vi "Main_Old.vi"() -> ()   [LabVIEW 2023]
uses:
  System states.ctl
  System variables.ctl
  <vilib>/Utility/file.llb/Read Delimited Spreadsheet (string).vi
  <vilib>/Utility/file.llb/Write Delimited Spreadsheet (string).vi
  Numato/Numato.lvlib
  DO_Reley/DO_Relay.lvlib
panel:
  in  "Tab Control":T1(tab)
  in  "Login":bool
  in  "Lozinka":string
  in  "Dostupne varijante":string(combo)
  in  "Select Variant":bool=TRUE
  in  "Izabrana varijanta":string
  in  "Cassete numbers":map{string, i32}(c390)
  out "Variants->FileNames":map{string, string}(c390)
  in  "Serial number":string
  in  "Report Erase":bool
  in  "START":bool
  in  "Status":bool[](array[boolean])
  in  "Stop":bool
  out "Monitor":string
  # "Rezultat brisanja programa :"
  # "Serisjki broj za brisanje :"
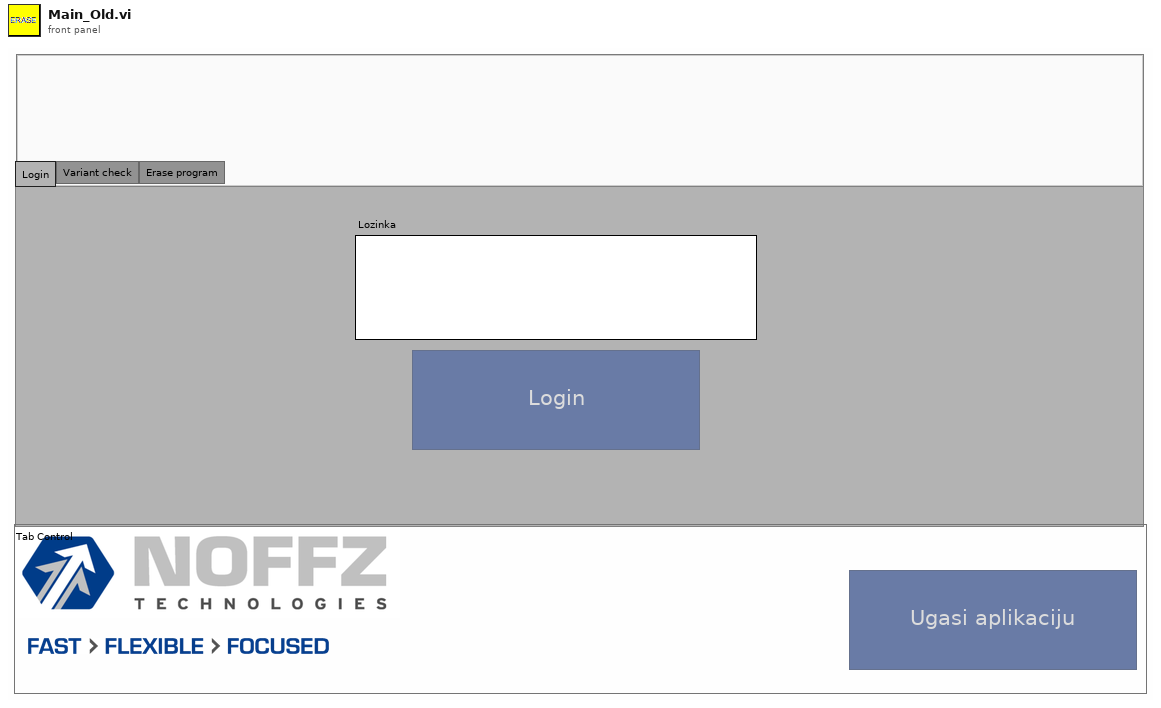
[diagram p1: front panel]
types:
  T1 = enum32{"Login", "Variant check", "Erase program"}
  T2 = typedef "System variables.ctl" = cluster{"Relay 1":refnum<visa-resource-name>, "Relay 2":refnum<visa-resource-name>, "Releji":cluster{"Vdd":i32, "GND":i32, "PGD":i32, "PGC":i32, "Reset":i32, "Reference":refnum<visa-resource-name>}, "DUT1":bool, "Family name":string, "DUT 2":bool, "DUT test?":bool, "DI0-7":i32, "DI8-15":i32, "DO0-8":i32, "References":cluster{"Relays":bool, "DIO":bool}}
  T3 = typedef "System states.ctl" = enum16{"Login", "Check Variant", "Dispaly variants", "Correct Variant", "Incorrect variant", "Initialize", "Check present boards", "Idle", "Connect relays", "Erasing", "Disconnect relays", "Erase Finished", "Deinitialize", "Erase report", "Set variables"}
  T4 = cluster{"Vdd":i32, "GND":i32, "PGD":i32, "PGC":i32, "Reset":i32, "Reference":refnum<visa-resource-name>}
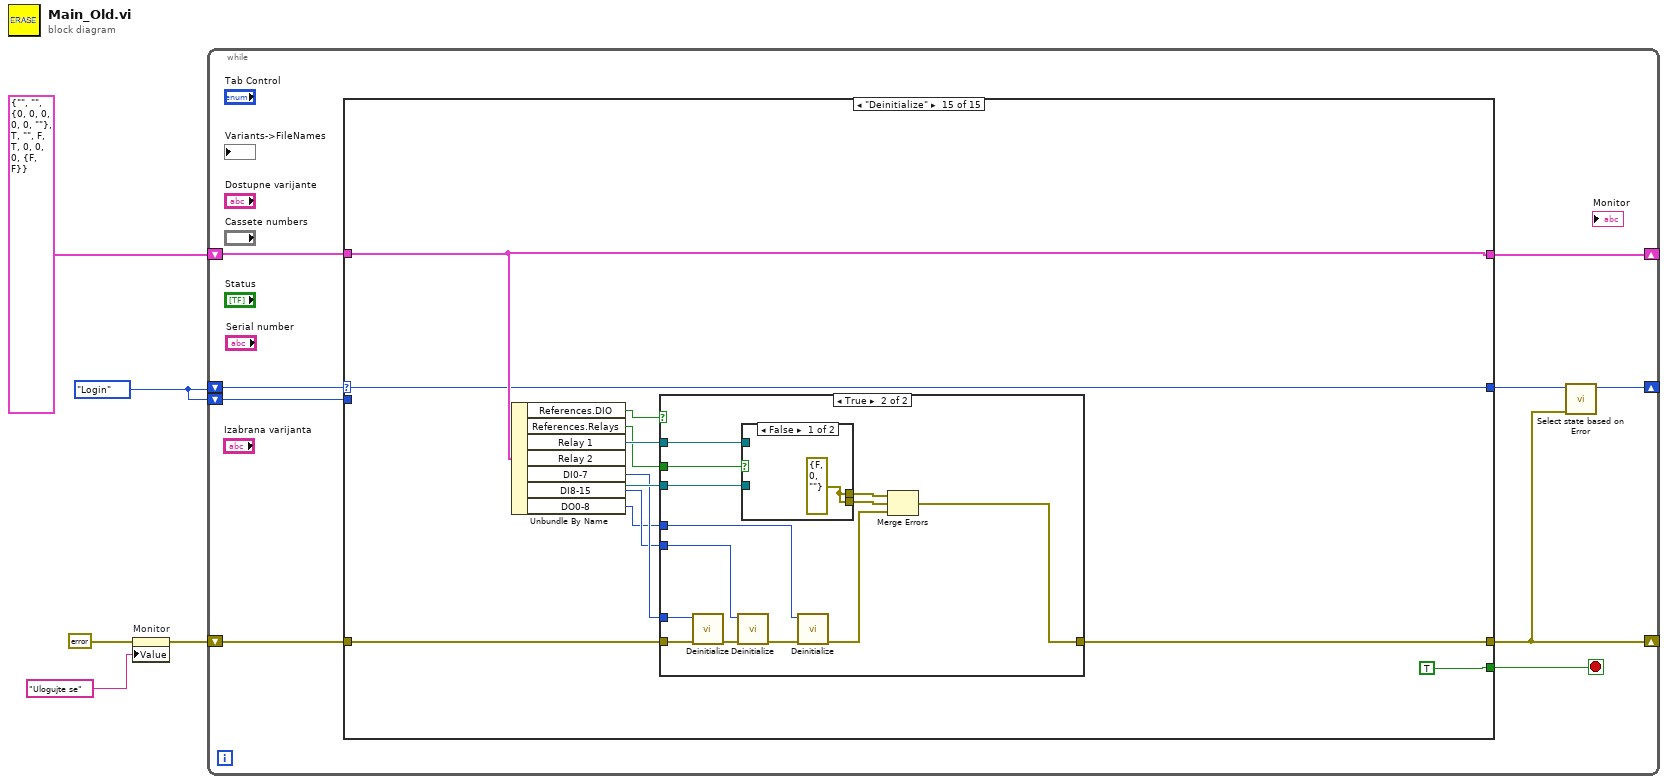
[diagram p0: block diagram]
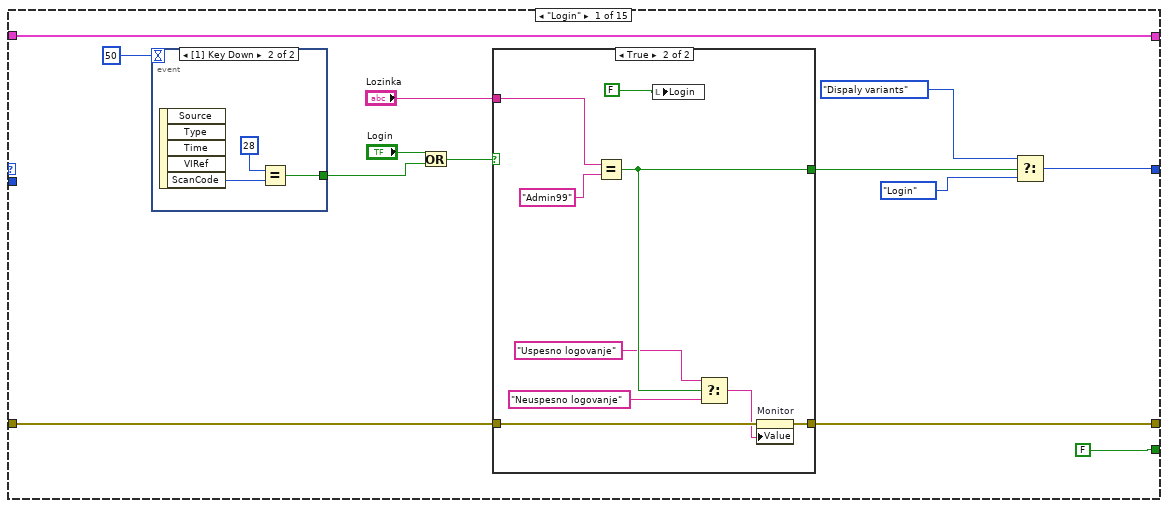
[diagram p2: hidden frame]
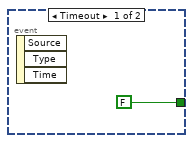
[diagram p3: hidden frame]
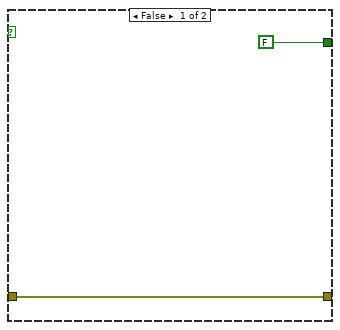
[diagram p4: hidden frame]
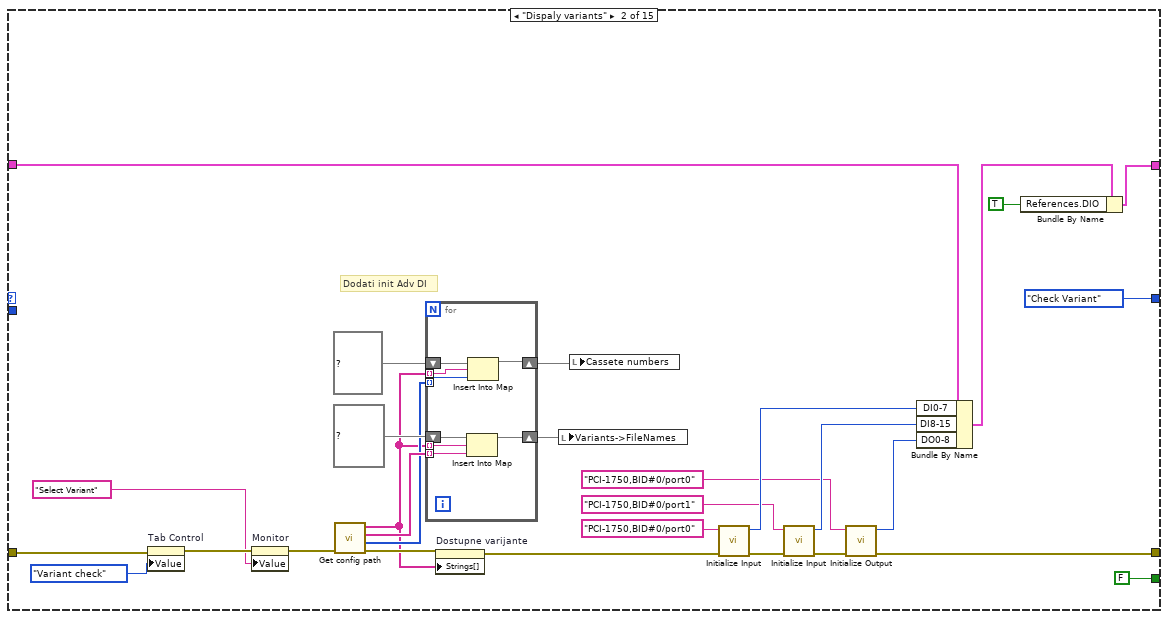
[diagram p5: hidden frame]
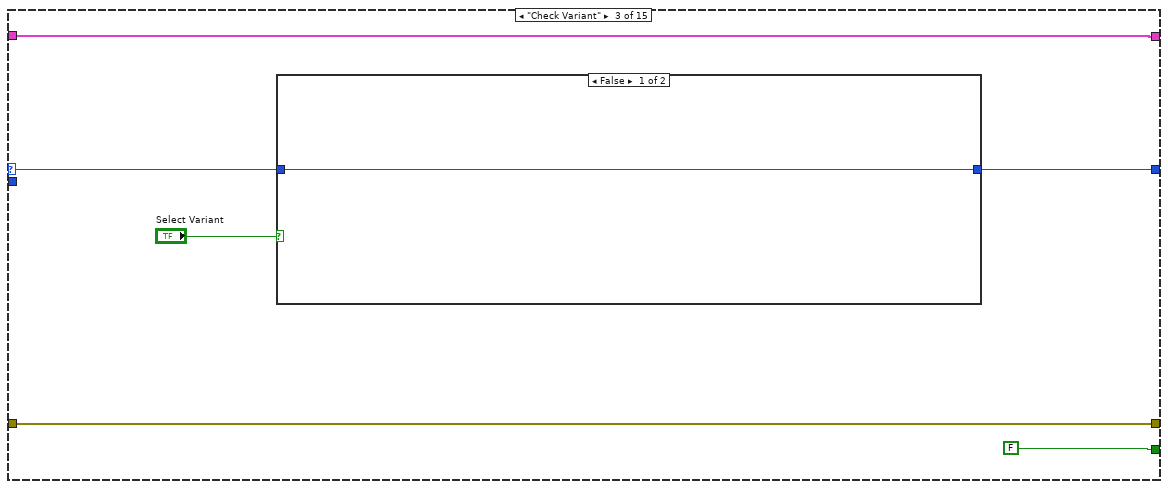
[diagram p6: hidden frame]
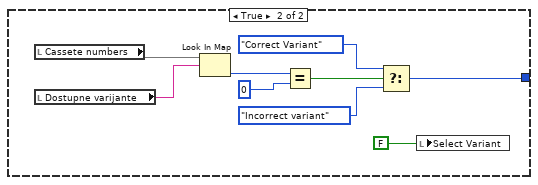
[diagram p7: hidden frame]
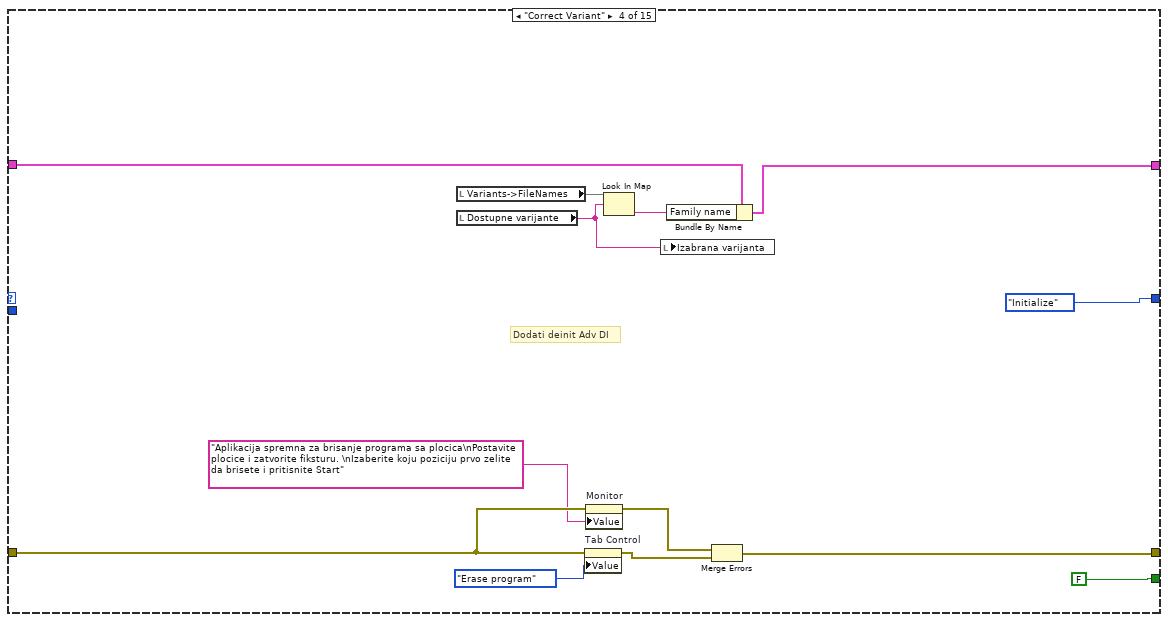
[diagram p8: hidden frame]
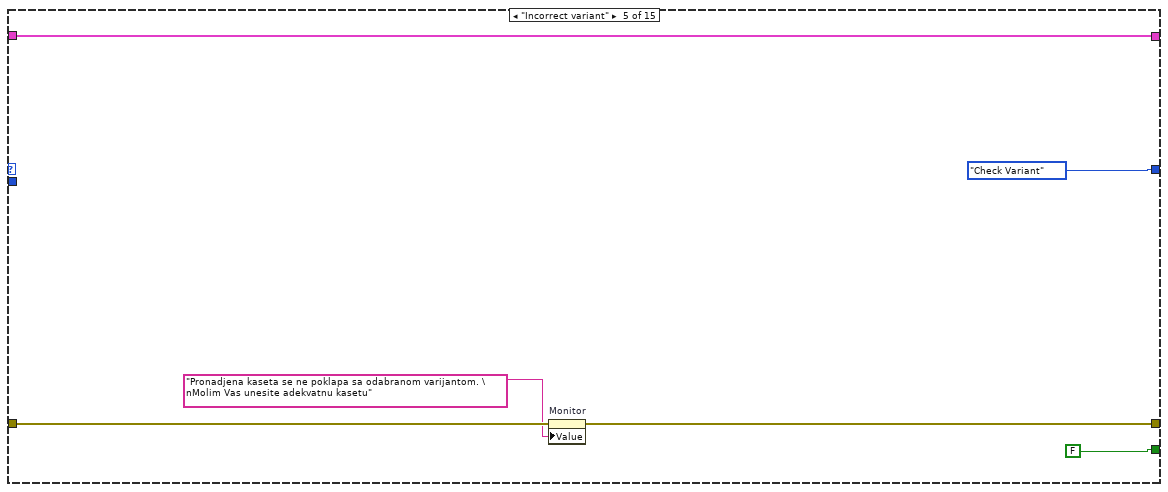
[diagram p9: hidden frame]
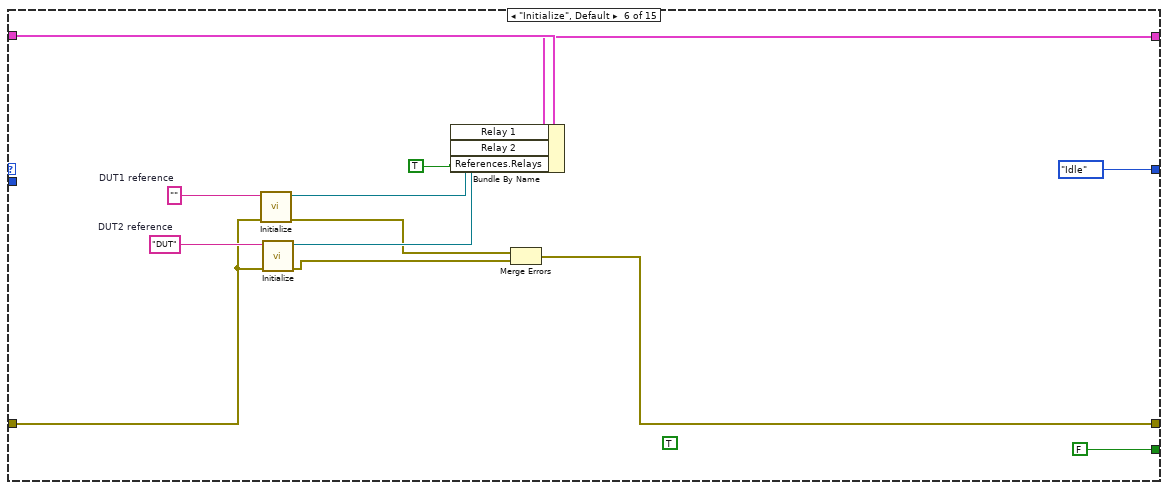
[diagram p10: hidden frame]
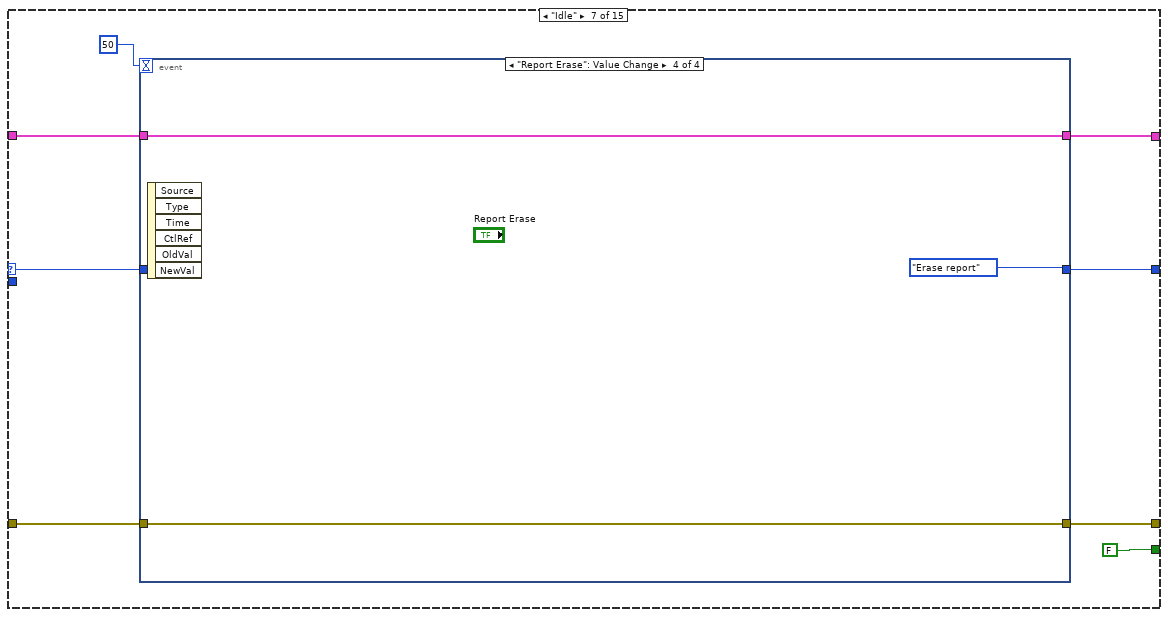
[diagram p11: hidden frame]
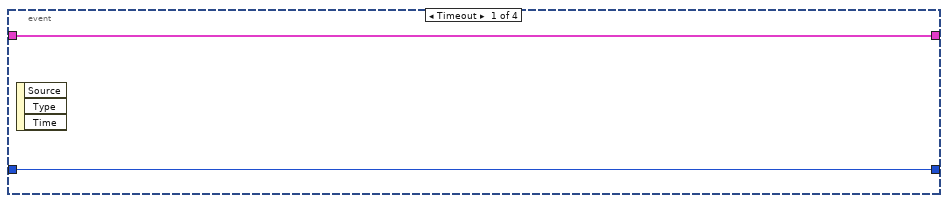
[diagram p12: hidden frame]
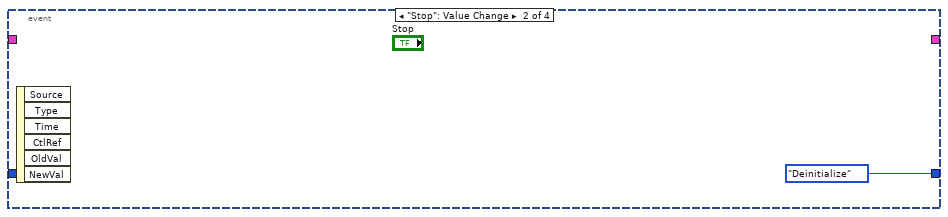
[diagram p13: hidden frame]
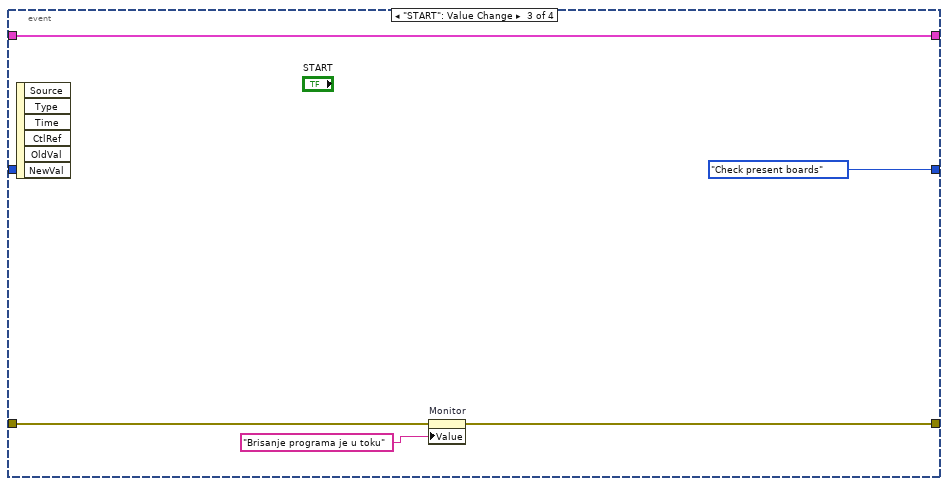
[diagram p14: hidden frame]
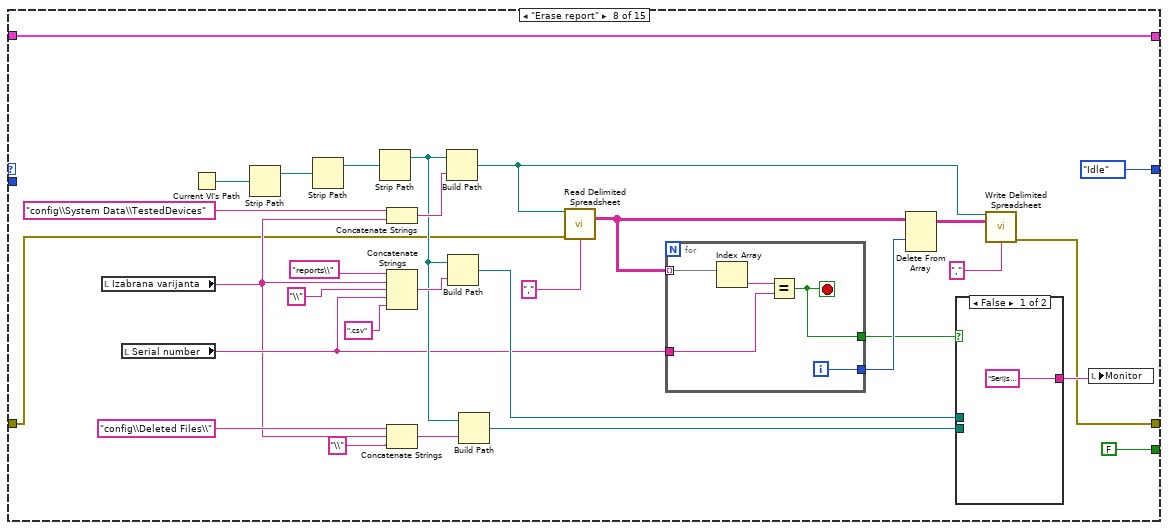
[diagram p15: hidden frame]
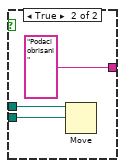
[diagram p16: hidden frame]
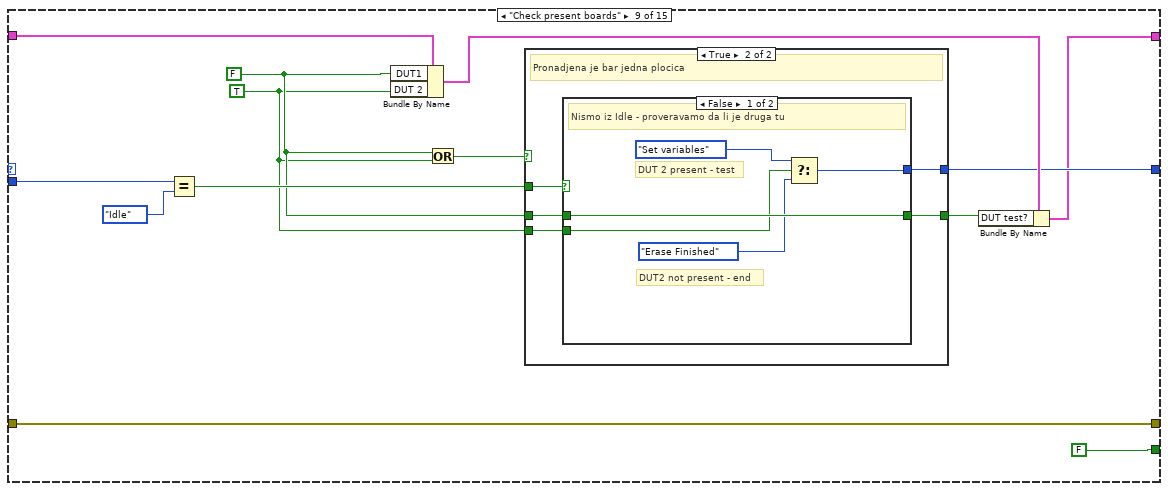
[diagram p17: hidden frame]
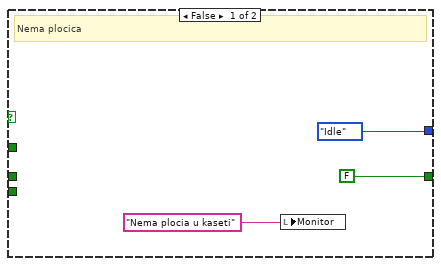
[diagram p18: hidden frame]
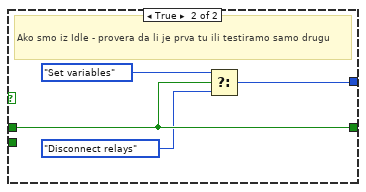
[diagram p19: hidden frame]
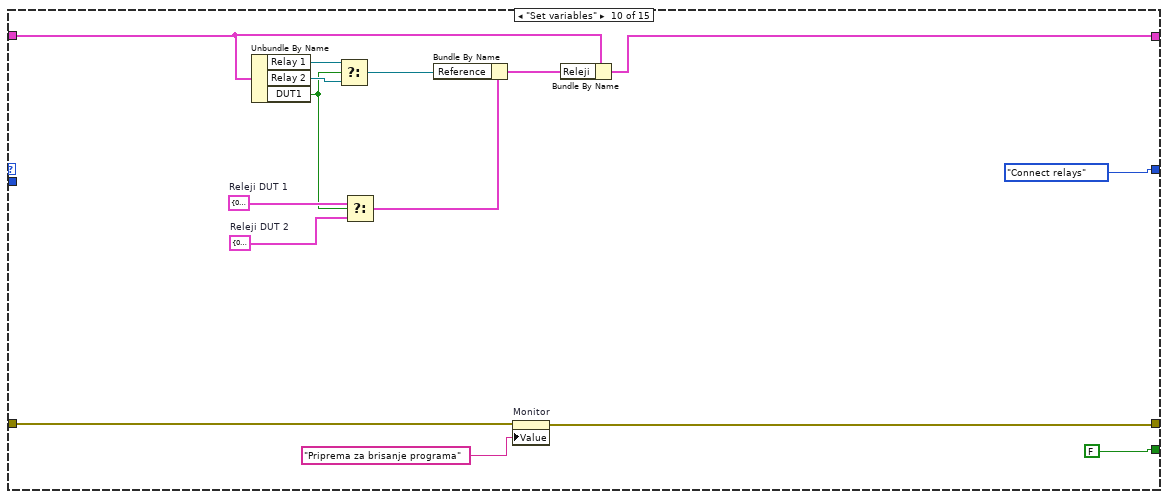
[diagram p20: hidden frame]
diagram:
  w1 = System_states."Login"
  n1 = property on="Monitor" class="Str"(error in=errorcluster {"status"=FALSE, "code"=0, "source"=""} ("error in (no error)"), "Value"="Ulogujte se" ("Monitor")) -> (error out=w3:errorcluster)  [unwired: 1 in, 1 out]
  n2 = while {
    shift-right: [w9] -> _
    shift-left: T2 {"Relay 1"="", "Relay 2"="", "Releji"={"Vdd"=0, "GND"=0, "PGD"=0, "PGC"=0, "Reset"=0, "Reference"=""}, "DUT1"=TRUE, "Family name"="", "DUT 2"=FALSE, "DUT test?"=TRUE, "DI0-7"=0, "DI8-15"=0, "DO0-8"=0, "References"={"Relays"=FALSE, "DIO"=FALSE}} -> [w13]
    shift-right: [w10] -> _
    shift-left: w3 -> [w14]
    shift-right: [w11] -> _
    shift-left: w1 -> [w7]
    shift-left: w1 -> [w6]
    stop <- w8 stop-if-true
    n3 = case shown="\"Deinitialize\"" w7 {
      selector: w7 -> [_ _ w84 _ _ _ w131 _ _ _ _ _ _ _ w278]
      tunnel: w14 -> [w21 w70 w82 w101 w114 w125 w129 w151 w195 w219 w235 w249 w262 w268 w276]
      tunnel: w13 -> [w15 w54 w80 w103 w111 w124 w134 w147 w198 w226 w234 w244 w259 w269 w280]
      tunnel: [w15 w44 w80 w102 w111 w123 w133 w147 w187 w230 w234 w244 w259 w269 w280] -> w9
      tunnel: [w20 w51 w82 w100 w113 w116 w128 w150 w195 w218 w236 w247 w261 w267 w275] -> w10
      tunnel: [w25 System_states."Check Variant" w83 System_states."Initialize" System_states."Check Variant" System_states."Idle" w132 System_states."Idle" w196 System_states."Connect relays" System_states."Erasing" System_states."Disconnect relays" w255 System_states."Idle" w278] -> w12
      tunnel: [FALSE ("Boolean") FALSE ("Boolean") FALSE ("Boolean") FALSE ("Boolean") FALSE ("Boolean") FALSE ("Boolean") FALSE ("Boolean") FALSE ("Boolean") FALSE ("Boolean") FALSE ("Boolean") FALSE ("Boolean") FALSE ("Boolean") FALSE ("Boolean") FALSE ("Boolean") TRUE ("Boolean")] -> w8
      tunnel: w6 -> [_ _ _ _ _ _ _ _ w193 _ _ _ _ _ _]
      frame "Login" {
        n4 = event shown="[1] Key Down" {
          selector: _ -> [_ _]
          dyn-events: _ -> [_ _]
          timeout: 50 -> [_ _]
          tunnel: [FALSE w29] -> w18
          event Timeout {
            n5 = event-data() -> ()  [unwired: 1 in, 3 out]
          }
          event Key Down {
            n6 = event-data() -> ("ScanCode"=w31:i16)  [unwired: 1 in, 4 out]
            n7 = Equal?(x=i16 28, y=w31) -> (x = y?=w29:bool)
          }
        }
        n8 = Or(x="Login", y=w18) -> (x .or. y?=w17:bool)
        n9 = case shown="True" w17 {
          tunnel: "Lozinka" -> [_ w42]
          tunnel: [FALSE w37] -> w22
          tunnel: w21 -> [w32 w39]
          tunnel: [w32 w38] -> w20
          frame False {
          }
          frame True {
            n10 = Equal?(x=w42, y="Admin99") -> (x = y?=w37:bool)
            n11 = local write "Login"(FALSE ("Login")) -> ()
            n12 = Select(t="Uspesno logovanje" ("y"), s=w37, f="Neuspesno logovanje" ("y")) -> (s? t:f=w34:string)
            n13 = property on="Monitor" class="Str"(error in=w39, "Value"=w34) -> (error out=w38:errorcluster)  [unwired: 1 in, 1 out]
          }
        }
        n14 = Select(t=System_states."Dispaly variants", s=w22, f=System_states."Login") -> (s? t:f=w25:T3)
      }
      frame "Dispaly variants" {
        # "Dodati init Adv DI"
        n15 = property on="Tab Control" class="TabCtl (strict)"(error in=w70, "Value"=T1."Variant check" ("Tab Control")) -> (error out=w68:errorcluster)  [unwired: 1 in, 1 out]
        n16 = property on="Monitor" class="Str"(error in=w68, "Value"="Select Variant" ("Monitor")) -> (error out=w66:errorcluster)  [unwired: 1 in, 1 out]
        n17 = call "Get config path.vi"("error in"=w66) -> ("error out"=w65:errorcluster, "Cassette codes"=w58:i32[], "Family names"=w64:string[], "Variants"=w57:string[])  [unwired: 7 in]
        n18 = for {
          tunnel: w57 -> [w77] mode=indexing
          tunnel: w64 -> [w76] mode=indexing
          shift-right: [w78] -> w61
          shift-left: map{string, string} {} ("Variants->FileNames") -> [w79]
          shift-right: [w74] -> w59
          shift-left: map{string, i32} {} ("map") -> [w75]
          tunnel: w57 -> [w73] mode=indexing
          tunnel: w58 -> [w72] mode=indexing
          n19 = Insert Into Map(map in=w79, key=w77, value=w76) -> (map out=w78:map{string, string})  [unwired: 2 out]
          n20 = Insert Into Map(map in=w75, key=w73, value=w72) -> (map out=w74:map{string, i32})  [unwired: 2 out]
        }
        n21 = property on="Dostupne varijante" class="CmbBox"(error in=w65, "Strings[]"=w57) -> (error out=w56:errorcluster)  [unwired: 1 in, 1 out]
        n22 = local write "Variants->FileNames"(w61) -> ()
        n23 = local write "Cassete numbers"(w59) -> ()
        n24 = call "Initialize Input.vi"("error in"=w56, "Physical channels in"="PCI-1750,BID#0/port0") -> ("error out"=w53:errorcluster, "task out"=w50:i32)  [unwired: 8 in]
        n25 = call "Initialize Input.vi"("error in"=w53, "Physical channels in"="PCI-1750,BID#0/port1") -> ("error out"=w52:errorcluster, "task out"=w49:i32)  [unwired: 8 in]
        n26 = call "Initialize Output.vi"("error in"=w52, "Physical channels in"="PCI-1750,BID#0/port0") -> ("error out"=w51:errorcluster, "task out"=w48:i32)  [unwired: 8 in]
        n27 = Bundle By Name(cluster=w54, "DI0-7"=w50, "DI8-15"=w49, "DO0-8"=w48) -> (w45:T2)
        n28 = Bundle By Name(cluster=w45, "References.DIO"=TRUE) -> (w44:T2)
      }
      frame "Check Variant" {
        n29 = case shown="False" "Select Variant" {
          tunnel: w84 -> [w86 _]
          tunnel: [w86 w93] -> w83
          frame False {
          }
          frame True {
            n30 = local read "Cassete numbers"() -> (w92:map{string, i32})
            n31 = local read "Dostupne varijante"() -> (w94:string)
            n32 = Look In Map(map=w92, key=w94) -> (value=w91:i32)  [unwired: 1 in, 1 out]
            n33 = Equal?(x=w91, y=0) -> (x = y?=w89:bool)
            n34 = Select(t=System_states."Correct Variant", s=w89, f=System_states."Incorrect variant") -> (s? t:f=w93:T3)
            n35 = local write "Select Variant"(FALSE ("Select Variant")) -> ()
          }
        }
      }
      frame "Correct Variant" {
        # "Dodati deinit Adv DI"
        n36 = local read "Variants->FileNames"() -> (w105:map{string, string})
        n37 = local read "Dostupne varijante"() -> (w96:string)
        n38 = property on="Tab Control" class="TabCtl (strict)"(error in=w101, "Value"=T1."Erase program" ("Tab Control")) -> (error out=w106:errorcluster)  [unwired: 1 in, 1 out]
        n39 = property on="Monitor" class="Str"(error in=w101, "Value"="Aplikacija spremna za brisanje programa sa plocica\nPostavite plocice i zatvorite fiksturu. \nIzaberite koju poziciju prvo zelite da brisete i pritisnite Start" ("Monitor")) -> (error out=w107:errorcluster)  [unwired: 1 in, 1 out]
        n40 = Look In Map(map=w105, key=w96) -> (value=w104:string)  [unwired: 1 in, 1 out]
        n41 = local write "Izabrana varijanta"(w96) -> ()
        n42 = Bundle By Name(cluster=w103, "Family name"=w104) -> (w102:T2)
        n43 = Merge Errors(w107, w106) -> (w100:errorcluster)
      }
      frame "Incorrect variant" {
        n44 = property on="Monitor" class="Str"(error in=w114, "Value"="Pronadjena kaseta se ne poklapa sa odabranom varijantom. \nMolim Vas unesite adekvatnu kasetu" ("Monitor")) -> (error out=w113:errorcluster)  [unwired: 1 in, 1 out]
      }
      frame "Initialize", Default {
        (unwired) TRUE ("DUT 1")
        w126 = ""  # DUT1 reference
        w127 = "DUT"  # DUT2 reference
        n45 = call "Initialize.vi"("error in (no error)"=w125, "Resource"=w126) -> ("error out"=w120:errorcluster, "VISA resource name out"=w122:refnum<visa-resource-name>)  [unwired: 8 in]
        n46 = call "Initialize.vi"("error in (no error)"=w125, "Resource"=w127) -> ("error out"=w119:errorcluster, "VISA resource name out"=w121:refnum<visa-resource-name>)  [unwired: 8 in]
        n47 = Bundle By Name(cluster=w124, "Relay 1"=w122, "Relay 2"=w121, "References.Relays"=TRUE) -> (w123:T2)
        n48 = Merge Errors(w120, w119) -> (w116:errorcluster)
      }
      frame "Idle" {
        n49 = event shown="[3] \"Report Erase\": Value Change" {
          selector: _ -> [_ _ _ _]
          dyn-events: _ -> [_ _ _ _]
          timeout: 50 -> [_ _ _ _]
          tunnel: w134 -> [w137 _ w142 w144]
          tunnel: [w137 _ w142 w144] -> w133
          tunnel: [w136 System_states."Deinitialize" System_states."Check present boards" System_states."Erase report"] -> w132
          tunnel: w131 -> [w136 _ _ _]
          tunnel: w129 -> [_ _ w141 w145]
          tunnel: [_ _ w140 w145] -> w128
          event Timeout {
            n50 = event-data() -> ()  [unwired: 1 in, 3 out]
          }
          event "Stop": Value Change {
            n51 = event-data() -> ()  [unwired: 1 in, 6 out]
          }
          event "START": Value Change {
            n52 = event-data() -> ()  [unwired: 1 in, 6 out]
            n53 = property on="Monitor" class="Str"(error in=w141, "Value"="Brisanje programa je u toku" ("Monitor")) -> (error out=w140:errorcluster)  [unwired: 1 in, 1 out]
          }
          event "Report Erase": Value Change {
            n54 = event-data() -> ()  [unwired: 1 in, 6 out]
          }
        }
      }
      frame "Erase report" {
        n55 = local read "Izabrana varijanta"() -> (w156:string)
        n56 = local read "Serial number"() -> (w158:string)
        n57 = Current VI's Path() -> (path=w174:path)
        n58 = Strip Path(path=w174) -> (stripped path=w175:path)  [unwired: 1 out]
        n59 = Strip Path(path=w175) -> (stripped path=w176:path)  [unwired: 1 out]
        n60 = Strip Path(path=w176) -> (stripped path=w163:path)  [unwired: 1 out]
        n61 = Concatenate Strings("config\\System Data\\TestedDevices", w156) -> (w172:string)
        n62 = Concatenate Strings("reports\\", w156, "\\" ("string"), w158, ".csv" ("string")) -> (w165:string)
        n63 = Concatenate Strings("config\\Deleted Files\\", w156, "\\" ("string")) -> (w161:string)
        n64 = Build Path(base path=w163, name or relative path=w172) -> (appended path=w167:path)
        n65 = Build Path(base path=w163, name or relative path=w165) -> (appended path=w164:path)
        n66 = Build Path(base path=w163, name or relative path=w161) -> (appended path=w154:path)
        n67 = call-poly <vilib>:"Read Delimited Spreadsheet.vi"("file path (dialog if empty)"=w167, "error in (no error)"=w151, "delimiter (\\t)"="," ("delimiter (\\t)")) -> ("all rows"=w170:string[][])  [unwired: 7 in, 5 out]
        n68 = for {
          tunnel: w170 -> [w185] mode=indexing
          tunnel: w158 -> [w183]
          tunnel: [w182] -> w169
          tunnel: [w181] -> w153
          i -> [w182]
          stop <- w181 stop-if-true
          n69 = Index Array(array=w185) -> (element=w184:string)  [unwired: 1 in]
          n70 = Equal?(x=w184, y=w183) -> (x = y?=w181:bool)
        }
        n71 = Delete From Array(array=w170, index (row)=w169) -> (array with subset deleted=w168:string[][])  [unwired: 2 in, 1 out]
        n72 = case shown="False" w153 {
          tunnel: w164 -> [_ w180]
          tunnel: w154 -> [_ w179]
          tunnel: ["Serijski broj nije pronajden u brojacu testiranja" ("Monitor") "Podaci obrisani" ("Monitor")] -> w152
          frame False {
          }
          frame True {
            n73 = Move(source path=w180, 10:w179) -> ()  [unwired: 3 in, 3 out]
          }
        }
        n74 = call-poly <vilib>:"Write Delimited Spreadsheet.vi"("file path (dialog if empty)"=w167, "2D data"=w168, "delimiter (\\t)"="," ("delimiter (\\t)")) -> ("error out"=w150:errorcluster)  [unwired: 11 in, 1 out]
        n75 = local write "Monitor"(w152) -> ()
      }
      frame "Check present boards" {
        w189 = FALSE ("DUT1")
        w188 = TRUE
        n76 = Equal?(x=w193, y=System_states."Idle") -> (x = y?=w191:bool)
        n77 = Bundle By Name(cluster=w198, "DUT1"=w189, "DUT 2"=w188) -> (w197:T2)
        n78 = Or(x=w189, y=w188) -> (x .or. y?=w190:bool)
        n79 = case shown="True" w190 {
          tunnel: [System_states."Idle" ("f") w206] -> w196
          tunnel: w191 -> [_ w205]
          tunnel: w189 -> [_ w204]
          tunnel: w188 -> [_ w203]
          tunnel: [FALSE ("DUT1") w202] -> w186
          frame False {
            # "Nema plocica"
            n80 = local write "Monitor"("Nema plocia u kaseti" ("Monitor")) -> ()
          }
          frame True {
            # "Pronadjena je bar jedna plocica"
            n81 = case shown="False" w205 {
              tunnel: [w208 w214] -> w206
              tunnel: w204 -> [w211 w215]
              tunnel: w203 -> [w210 _]
              tunnel: [w211 w215] -> w202
              frame False {
                # "DUT2 not present - end"
                # "DUT 2 present - test"
                # "Nismo iz Idle - proveravamo da li je druga tu"
                n82 = Select(t=System_states."Set variables", s=w210, f=System_states."Erase Finished") -> (s? t:f=w208:T3)
              }
              frame True {
                # "Ako smo iz Idle - provera da li je prva tu ili testiramo samo drugu"
                n83 = Select(t=System_states."Set variables" ("f"), s=w215, f=System_states."Disconnect relays") -> (s? t:f=w214:T3)
              }
            }
          }
        }
        n84 = Bundle By Name(cluster=w197, "DUT test?"=w186) -> (w187:T2)
      }
      frame "Set variables" {
        w228 = T4 {"Vdd"=0, "GND"=0, "PGD"=0, "PGC"=0, "Reset"=0, "Reference"=""}  # Releji DUT 2
        w229 = T4 {"Vdd"=0, "GND"=0, "PGD"=0, "PGC"=0, "Reset"=0, "Reference"=""}  # Releji DUT 1
        n85 = Unbundle By Name(w226) -> ("Relay 1"=w225:refnum<visa-resource-name>, "Relay 2"=w224:refnum<visa-resource-name>, "DUT1"=w220:bool)
        n86 = Select(t=w225, s=w220, f=w224) -> (s? t:f=w223:refnum<visa-resource-name>)
        n87 = Select(t=w229, s=w220, f=w228) -> (s? t:f=w227:T4)
        n88 = Bundle By Name(cluster=w227, "Reference"=w223) -> (w222:T4)
        n89 = property on="Monitor" class="Str"(error in=w219, "Value"="Priprema za brisanje programa" ("Monitor")) -> (error out=w218:errorcluster)  [unwired: 1 in, 1 out]
        n90 = Bundle By Name(cluster=w226, "Releji"=w222) -> (w230:T2)
      }
      frame "Connect relays" {
        # "Lock fixture"
        n91 = call "Set relays.vi"("error in (no error)"=w235, "System Variables"=w234, "ON/OFF"=TRUE) -> ("error out"=w236:errorcluster)  [unwired: 8 in]
      }
      frame "Erasing" {
        w252 = TRUE  # Supply PCB over Programator
        w254 = FALSE  # 6.25
        n92 = Unbundle By Name(w244) -> ("DUT1"=w241:bool, "Family name"=w253:string)
        n93 = property on="Monitor" class="Str"(error in=w249, "Value"="Brisanje programa je u toku" ("Monitor")) -> (error out=w246:errorcluster)  [unwired: 1 in, 1 out]
        n94 = call "Erase Memory.vi"("DUT1?"=w241, "error in"=w249, "Supply PCB over Programator"=w252, "Family"=w253, "6.25"=w254) -> ("error out"=w248:errorcluster, "Erase passed"=w237:bool)  [unwired: 3 in, 2 out]
        n95 = Select(t=0 ("index"), s=w241, f=1 ("index")) -> (s? t:f=w239:i32)
        n96 = local read "Status"() -> (w243:bool[])
        n97 = Merge Errors(w248, w246) -> (w247:errorcluster)
        n98 = Replace Array Subset(array=w243, new element=w237, index=w239) -> (w242:bool[])
        n99 = local write "Status"(w242) -> ()
      }
      frame "Disconnect relays" {
        # "If DUT2 was tested - No need to test more\ncontinue to end"
        # "DUT1 is tested first - if this was DUT1 then\ngo back to test DUT2 if present"
        # "unlock fixture"
        n100 = call "Set relays.vi"("error in (no error)"=w262, "System Variables"=w259, "ON/OFF"=FALSE) -> ("error out"=w261:errorcluster)  [unwired: 8 in]
        n101 = Unbundle By Name(w259) -> ("DUT test?"=w257:bool)
        n102 = Select(t=System_states."Check present boards", s=w257, f=System_states."Erase Finished") -> (s? t:f=w255:T3)
      }
      frame "Erase Finished" {
        n103 = property on="Monitor" class="Str"(error in=w268, "Value"="Brisanje programa je gotovo\nStanica je spremna za narednu plocice" ("Monitor")) -> (error out=w267:errorcluster)  [unwired: 1 in, 1 out]
      }
      frame "Deinitialize" {
        n104 = Unbundle By Name(w280) -> ("References.DIO"=w273:bool, "References.Relays"=w274:bool, "Relay 1"=w277:refnum<visa-resource-name>, "Relay 2"=w281:refnum<visa-resource-name>, "DI0-7"=w272:i32, "DI8-15"=w271:i32, "DO0-8"=w270:i32)
        n105 = case shown="True" w273 {
          tunnel: w281 -> [_ w295]
          tunnel: w277 -> [_ w294]
          tunnel: w276 -> [w282 w289]
          tunnel: [w282 w291] -> w275
          tunnel: w274 -> [_ w290]
          tunnel: w272 -> [_ w285]
          tunnel: w271 -> [_ w284]
          tunnel: w270 -> [_ w283]
          frame False {
          }
          frame True {
            n106 = call "Deinitialize.vi"("error in"=w289, "task in"=w285) -> ("error out"=w288:errorcluster)  [unwired: 9 in]
            n107 = call "Deinitialize.vi"("error in"=w288, "task in"=w284) -> ("error out"=w287:errorcluster)  [unwired: 9 in]
            n108 = case shown="False" w290 {
              tunnel: w295 -> [_ w300]
              tunnel: w294 -> [_ w299]
              tunnel: [w296 w298] -> w293
              tunnel: [w296 w297] -> w292
              frame False {
                w296 = errorcluster {"status"=FALSE, "code"=0, "source"=""} ("error out")
              }
              frame True {
                n109 = call "Deinitialize.vi"("VISA resource name"=w300) -> ("error out"=w297:errorcluster)  [unwired: 10 in]
                n110 = call "Deinitialize.vi"("VISA resource name"=w299) -> ("error out"=w298:errorcluster)  [unwired: 10 in]
              }
            }
            n111 = call "Deinitialize.vi"("error in"=w287, "task in"=w283) -> ("error out"=w286:errorcluster)  [unwired: 9 in]
            n112 = Merge Errors(w293, w292, w286) -> (w291:errorcluster)
          }
        }
      }
    }
    n113 = call "Select state based on Error.vi"("error in (no error)"=w10, "Wanted state"=w12) -> ("Next State"=w11:T3)  [unwired: 9 in]
  }
